vi "Uframe-MNR.vi"() -> ()   [LabVIEW 2010]
uses:
  <vilib>/Platform/TimedLoop/XDataNode/XDataNode.xnode
  <vilib>/Platform/TimedLoop/XDataNode/timing_clust.ctl
  <vilib>/Platform/TimedLoop/XDataNode/nitl_modes.ctl
  <vilib>/Platform/TimedLoop/XDataNode/wakeup.ctl
  <vilib>/Platform/TimedLoop/XDataNode/XDNodeRunTimeDep.lvlib
panel:
  out "Load Cell Constant (N/V)":dbl=44.48
  in  "Load Cell":u16(ring)=1 items=["440 N", "1250 N"]
  in  "Pause @ Load":bool
  in  "Pause @ N":dbl
  out "Disp (mm)":dbl
  out "Load (N)":dbl
  out "Data Point":i32
  in  "Max Load (N)":dbl=600.0 min=0.0 max=1200.0
  out "At Limit":bool
  in  "Rate Multiplier":dbl=1.0
  in  "Pause \nDisplacement":bool
  in  "Stop":bool
  in  "Invert \nDisplacement":bool
  in  "Zero \nDisplacement":bool=TRUE
  in  "Begin":bool
  out "Load vs Disp":cluster{dbl[], dbl[]}(graph)={[-724.1250113144533, -724.195323815552, -724.2656363166506, -724.3359488177492, -724.4062613188479, -724.4765738199465, -724.5468863210451, -724.6171988221438, -724.7461050741579, -724.9218863269045, -725.0976675796511, -725.2851675825808, -725.4492300851442], [-11.89350874713131, -11.896152101474941, -11.894229661847117, -11.89350874707076, -11.890865392620372, -11.895671491596438, -11.895911796524977, -11.899756675680168, -11.899035760801853, -11.90552399441818, -11.907927043887174, -11.905283689458143, -11.914655582386047]}
  out "Disp Vs Time":cluster{dbl[], dbl[]}(graph)={[-724.1250113144533, -724.195323815552, -724.2656363166506, -724.3359488177492, -724.4062613188479, -724.4765738199465, -724.5468863210451, -724.6171988221438, -724.7461050741579, -724.9218863269045, -725.0976675796511, -725.2851675825808, -725.4492300851442], [-11.89350874713131, -11.896152101474941, -11.894229661847117, -11.89350874707076, -11.890865392620372, -11.895671491596438, -11.895911796524977, -11.899756675680168, -11.899035760801853, -11.90552399441818, -11.907927043887174, -11.905283689458143, -11.914655582386047]}
  in  "File Name":string="Test"
  in  "File Path":path=path "C:/cygwin/home/Smarter Materials/Users 2015/Michael Rossol"
  in  "Sample Notes":string
  in  "Displacement \nRate (um/s)":dbl=3.0 min=3.0 max=50.0
  in  "Data Acquisition \nInterval (s)":dbl=1.0 min=0.1 max=10.0 step=0.01 format="%#_3g"
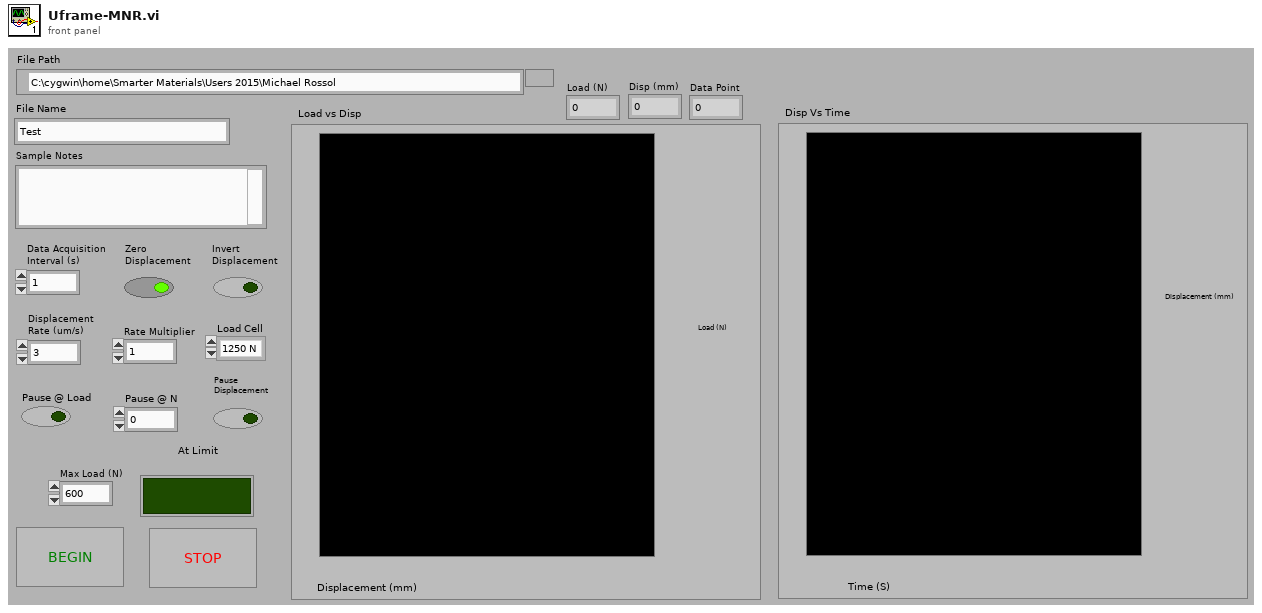
[diagram p1: front panel]
types:
  T1 = typedef "XDNodeRunTimeDep.lvlib/timing_clust.ctl" = cluster{"Expected End [f-1]":u64, "Actual End [f-1]":u64, "Finished Late? [f-1]":bool, "Expected End [i-1]":u64, "Actual End [i-1]":u64, "Finished Late? [i-1]":bool, "Expected Start [i]":u64, "Actual Start [i]":u64, "Expected Start [f]":u64, "Actual Start [f]":u64, "Source Name":string, "Structure Name":string, "Period":i64, "Deadline":i64, "Offset":i64, "Start":i64, "Priority":i32, "Timeout":i32, "Mode":T2, "Wakeup Reason":T3, "Error":errorcluster, "Source Type":string, "Secondary Source Type":string, "Global End Time":u64, "Global Start Time":u64, "Frame Duration":u64, "Iteration Duration":u64, "Assigned CPU":i32, "I/O Scan Engine Mode":u32}
  T2 = typedef "XDNodeRunTimeDep.lvlib/nitl_modes.ctl" = enum32{"No Change", "Process missed periods, maintain original phase", "Discard missed periods, maintain original phase", "Process missed periods, ignore original phase", "Discard missed periods, ignore original phase"}
  T3 = typedef "XDNodeRunTimeDep.lvlib/wakeup.ctl" = enum32{"Normal", "Aborted", "Asynchronous wakeup", "Timing source error", "Timed loop error", "Timeout"}
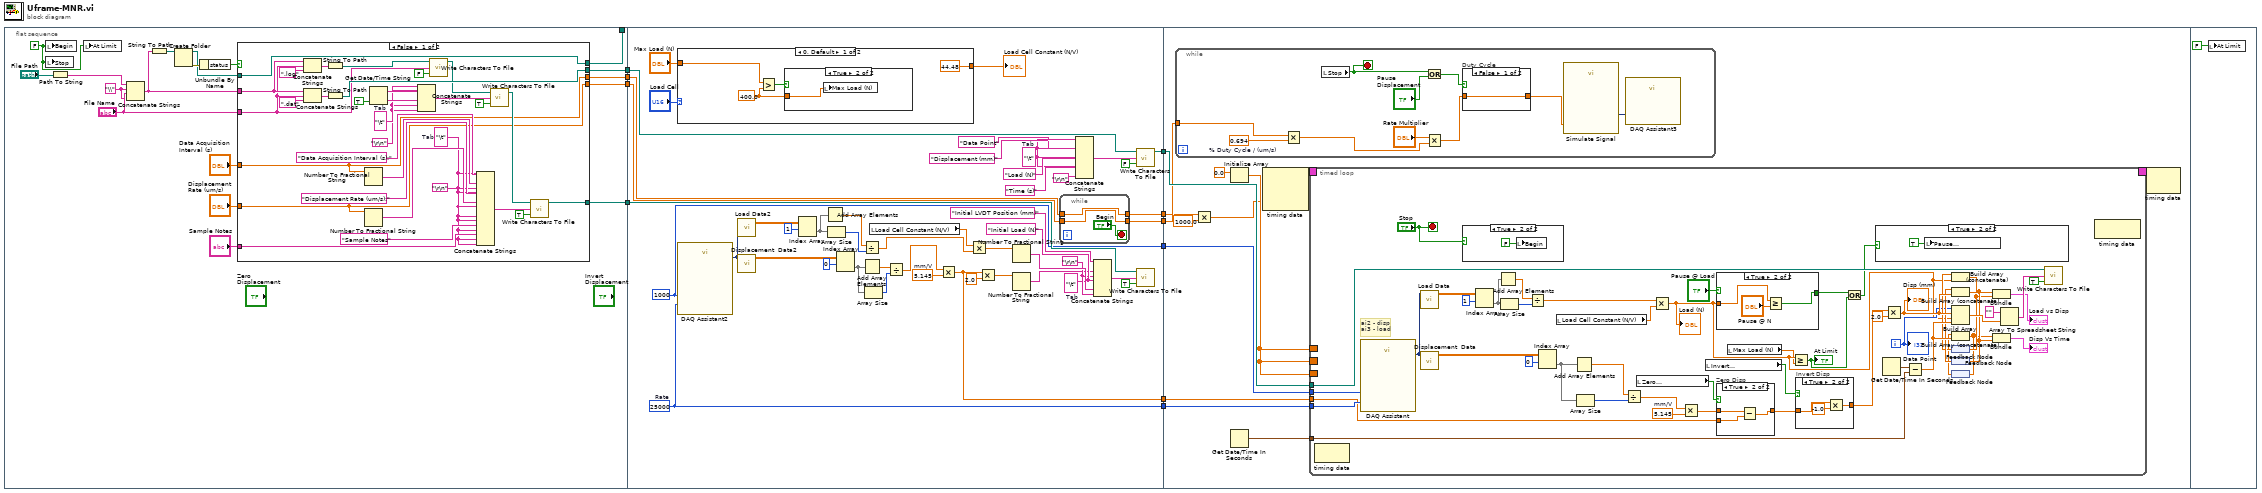
[diagram p0: block diagram]
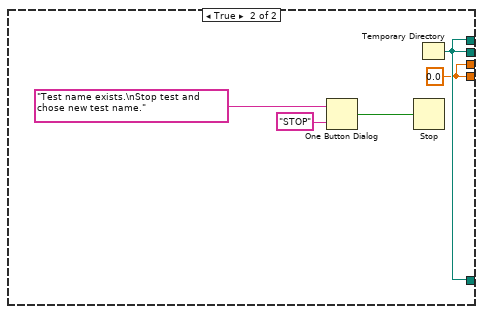
[diagram p2: hidden frame]
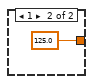
[diagram p4: hidden frame]
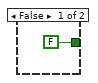
[diagram p5: hidden frame]
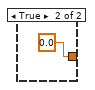
[diagram p10: hidden frame]
diagram:
  n1 = flat-sequence {
    tunnel: [w15] -> w6
    tunnel: [w27] -> w4
    tunnel: [w16] -> w3
    tunnel: [w17] -> w1
    tunnel: [w13] -> _
    tunnel: [w70] -> w10
    tunnel: [w71] -> w9
    tunnel: [w72] -> w8
    tunnel: [w77] -> w7
    tunnel: w6 -> [w91]
    tunnel: [w82] -> w5
    tunnel: w4 -> [w81]
    tunnel: w3 -> [w74]
    tunnel: [w73] -> w2
    tunnel: w1 -> [w75]
    tunnel: w10 -> [w123]
    tunnel: w9 -> [w134]
    tunnel: w8 -> [w133]
    tunnel: w7 -> [w132]
    tunnel: w5 -> [w131]
    tunnel: w2 -> [w130]
    frame #0 {
      w14 = FALSE ("Begin")
      w12 = "\\"
      n2 = local write "Begin"(w14) -> ()
      n3 = local write "Stop"(w14) -> ()
      n4 = Path To String(path="File Path") -> (string=w22:string)
      n5 = local write "At Limit"(w14) -> ()
      n6 = Concatenate Strings(w22, w12, "File Name", w12) -> (w20:string)
      n7 = String To Path(string=w20) -> (path=w24:path)
      n8 = Create Folder(path (use dialog)=w24) -> (created path=w11:path, error out=w23:errorcluster)  [unwired: 2 in, 1 out]
      n9 = Unbundle By Name(w23) -> ("status"=w21:bool)
      n10 = case shown="False" w21 {
        tunnel: [w46 w62] -> w15
        tunnel: "Data Acquisition \nInterval (s)" -> [w41 _]
        tunnel: "Displacement \nRate (um/s)" -> [w42 _]
        tunnel: "Sample Notes" -> [w38 _]
        tunnel: [w43 w62] -> w27
        tunnel: [w42 w61] -> w16
        tunnel: [w41 w61] -> w17
        tunnel: w20 -> [w31 _]
        tunnel: "File Name" -> [w30 _]
        tunnel: [w29 w62] -> w13
        tunnel: w11 -> [w29 _]
        frame False {
          w40 = "\t"  # Tab
          w37 = "\r\n"
          w56 = "\t"  # Tab
          w51 = "\r\n"
          n11 = Concatenate Strings(w31, w30, ".log") -> (w33:string)
          n12 = Concatenate Strings(w31, w30, ".dat") -> (w44:string)
          n13 = String To Path(string=w33) -> (path=w32:path)
          n14 = String To Path(string=w44) -> (path=w43:path)
          n15 = Number To Fractional String(number=w41) -> (F-format string=w49:string)  [unwired: 3 in]
          n16 = Number To Fractional String(number=w42) -> (F-format string=w47:string)  [unwired: 3 in]
          n17 = Get Date/Time String(want seconds? (F)=TRUE) -> (date string=w59:string, time string=w58:string)  [unwired: 2 in]
          n18 = Concatenate Strings(w51, w59, w56, w58, w51, w51) -> (w60:string)
          n19 = call <vilib>:"Write Characters To File.vi"("append to file? (new file:F)"=FALSE, "character string"=w30, "file path (dialog if empty)"=w32) -> ("new file path (Not A Path if cancelled)"=w36:path)  [unwired: 2 in]
          n20 = Concatenate Strings("Data Acquisition Interval (s):", w40, w49, w37, "Displacement Rate (um/s):", w40, w47, w37, w40, w37, w37, "Sample Notes", w37, w38, w37, w37) -> (w52:string)
          n21 = call <vilib>:"Write Characters To File.vi"("append to file? (new file:F)"=TRUE, "character string"=w60, "file path (dialog if empty)"=w36) -> ("new file path (Not A Path if cancelled)"=w54:path)  [unwired: 2 in]
          n22 = call <vilib>:"Write Characters To File.vi"("append to file? (new file:F)"=TRUE, "character string"=w52, "file path (dialog if empty)"=w54) -> ("new file path (Not A Path if cancelled)"=w46:path)  [unwired: 2 in]
        }
        frame True {
          w61 = 0.0 ("Displacement Rate (um/s)")
          n23 = One Button Dialog(message="Test name exists.\nStop test and chose new test name.", button name ("OK")="STOP") -> (true=w63:bool)
          n24 = Stop(stop? (T)=w63) -> ()
          n25 = Temporary Directory() -> (w62:path)
        }
      }
    }
    frame #1 {
      w72 = 1000 ("number of samples")
      w84 = "\t"  # Tab
      w95 = "\r\n"
      w93 = "\t"  # Tab
      w109 = 5.145  # mm/V
      w71 = 25000  # Rate
      n26 = case shown="0, Default" "Load Cell" {
        tunnel: [44.48 125.0] -> w68
        tunnel: "Max Load (N)" -> [w114 _]
        frame 0, Default {
          w113 = 400.0 ("y")
          n27 = Greater?(x=w114, y=w113) -> (0:w115:bool)
          n28 = case shown="True" w115 {
            tunnel: w113 -> [_ w117]
            frame False {
            }
            frame True {
              n29 = local write "Max Load (N)"(w117) -> ()
            }
          }
        }
        frame 1 {
        }
      }
      "Load Cell Constant (N/V)" <- w68
      n30 = call "DAQ Assistant2"("rate"=w71, "number of samples"=w72) -> ("data"=w100:dynamicdata)  [unwired: 15 in, 2 out]
      n31 = call "Load Data2"("Dynamic Data Type"=w100) -> ("Array"=w101:dbl[][])  [unwired: 3 in]
      n32 = call "Displacement  Data2"("Dynamic Data Type"=w100) -> ("Array"=w104:dbl[][])  [unwired: 3 in]
      n33 = Index Array(array=w101, index (row)=1) -> (element=w112:dbl[])  [unwired: 1 in]
      n34 = Add Array Elements(numeric array=w112) -> (sum=w110:dbl)
      n35 = Array Size(array=w112) -> (size(s)=w111:i32)
      n36 = Index Array(array=w104, index (row)=0) -> (element=w105:dbl[])  [unwired: 1 in]
      n37 = Divide(x=w110, y=w111) -> (x/y=w79:dbl)
      n38 = Add Array Elements(numeric array=w105) -> (sum=w106:dbl)
      n39 = Array Size(array=w105) -> (size(s)=w107:i32)
      n40 = local read "Load Cell Constant (N/V)"() -> (w69:dbl)
      n41 = Divide(x=w106, y=w107) -> (x/y=w108:dbl)
      n42 = Multiply(x=w108, y=w109) -> (x*y=w77:dbl)
      n43 = Multiply(x=w69, y=w79) -> (x*y=w80:dbl)
      n44 = Multiply(x=w77, y=2.0) -> (x*y=w78:dbl)
      n45 = Number To Fractional String(number=w80) -> (F-format string=w97:string)  [unwired: 3 in]
      n46 = Number To Fractional String(number=w78) -> (F-format string=w94:string)  [unwired: 3 in]
      n47 = while {
        tunnel: w74 -> [w120]
        tunnel: [w120] -> w73
        tunnel: [w119] -> w70
        tunnel: w75 -> [w119]
        stop <- "Begin" stop-if-true
      }
      n48 = Concatenate Strings("Data Point", w84, "Displacement (mm)" ("Substring"), w84, "Load (N)", w84, "Time (s)" ("string"), w84, "\r\n") -> (w89:string)
      n49 = Concatenate Strings("Initial LVDT Position (mm)", w93, w94, w95, "Initial Load (N)", w93, w97, w95) -> (w98:string)
      n50 = call <vilib>:"Write Characters To File.vi"("append to file? (new file:F)"=FALSE, "character string"=w89, "file path (dialog if empty)"=w81) -> ("new file path (Not A Path if cancelled)"=w82:path)  [unwired: 2 in]
      n51 = call <vilib>:"Write Characters To File.vi"("append to file? (new file:F)"=TRUE, "character string"=w98, "file path (dialog if empty)"=w91) -> ()  [unwired: 2 in, 1 out]
    }
    frame #2 {
      n52 = while {
        tunnel: w130 -> [w211]
        stop <- w204 stop-if-true
        w205 = 0.694  # % Duty Cycle / (um/s)
        n53 = Multiply(x=w211, y=w205) -> (x*y=w208:dbl)
        n54 = local read "Stop"() -> (w204:bool)
        n55 = Or(x=w204, y="Pause \nDisplacement") -> (x .or. y?=w210:bool)
        n56 = Multiply(x="Rate Multiplier", y=w208) -> (x*y=w207:dbl)
        n57 = case "Duty Cycle" shown="False" w210 {
          tunnel: [w214 0.0 ("Duty Cycle (%)")] -> w212
          tunnel: w207 -> [w214 _]
          frame False {
          }
          frame True {
          }
        }
        n58 = call "Simulate Signal"("Duty Cycle (%)"=w212) -> ("Square"=w213:dynamicdata)  [unwired: 13 in, 1 out]
        n59 = call "DAQ Assistant3"("data"=w213) -> ()  [unwired: 16 in, 3 out]
      }
      n60 = Multiply(x=w123, y=1000.0) -> (x*y=w124:dbl)
      n61 = Get Date/Time In Seconds() -> (seconds since 1Jan1904=w127:timestamp)
      n62 = Initialize Array(0.0) -> (w128:dbl[])  [unwired: 1 in]
      n63 = node-c288(w124) -> (w126:T1)  [unwired: 2 in]
      n64 = timed-loop {
        tunnel: w133 -> [w166]
        tunnel: w134 -> [w165]
        tunnel: w132 -> [w157]
        tunnel: w127 -> [w161]
        tunnel: w131 -> [w160]
        border: w128 -> [_]
        border: w128 -> [_]
        border: w128 -> [_]
        timing: w126 -> [_]
        timing-out: [_] -> w125
        i -> [w143]
        stop <- "Stop" stop-if-true
        w164 = 5.145  # mm/V
        # "ai2 - disp\nai3 - load"
        n65 = node-c288() -> ()  [unwired: 1 in, 1 out]
        n66 = call "DAQ Assistant"("rate"=w165, "number of samples"=w166) -> ("data"=w163:dynamicdata)  [unwired: 15 in, 2 out]
        n67 = call "Load Data"("Dynamic Data Type"=w163) -> ("Array"=w178:dbl[][])  [unwired: 3 in]
        n68 = call "Displacement  Data"("Dynamic Data Type"=w163) -> ("Array"=w175:dbl[][])  [unwired: 3 in]
        n69 = case shown="True" "Stop" {
          frame False {
          }
          frame True {
            n70 = local write "Begin"(FALSE ("Begin")) -> ()
          }
        }
        n71 = Index Array(array=w178, index (row)=1) -> (element=w167:dbl[])  [unwired: 1 in]
        n72 = Add Array Elements(numeric array=w167) -> (sum=w169:dbl)
        n73 = Array Size(array=w167) -> (size(s)=w168:i32)
        n74 = Divide(x=w169, y=w168) -> (x/y=w154:dbl)
        n75 = Index Array(array=w175, index (row)=0) -> (element=w173:dbl[])  [unwired: 1 in]
        n76 = local read "Load Cell Constant (N/V)"() -> (w136:dbl)
        n77 = Add Array Elements(numeric array=w173) -> (sum=w172:dbl)
        n78 = Array Size(array=w173) -> (size(s)=w171:i32)
        n79 = Divide(x=w172, y=w171) -> (x/y=w170:dbl)
        n80 = local read "Zero \nDisplacement"() -> (w155:bool)
        n81 = Multiply(x=w154, y=w136) -> (x*y=w138:dbl)
        "Load (N)" <- w138
        n82 = Multiply(x=w170, y=w164) -> (x*y=w159:dbl)
        n83 = local read "Invert \nDisplacement"() -> (w156:bool)
        n84 = case shown="True" "Pause @ Load" {
          tunnel: w138 -> [_ w186]
          tunnel: [FALSE w185] -> w137
          frame False {
          }
          frame True {
            n85 = Greater Or Equal?(x=w186, y="Pause @ N") -> (x >= y?=w185:bool)
          }
        }
        n86 = case "Zero Disp" shown="True" w155 {
          tunnel: w157 -> [_ w199]
          tunnel: w159 -> [w196 w198]
          tunnel: [w196 w197] -> w158
          frame False {
          }
          frame True {
            n87 = Subtract(x=w198, y=w199) -> (x-y=w197:dbl)
          }
        }
        n88 = local read "Max Load (N)"() -> (w135:dbl)
        n89 = Greater Or Equal?(x=w138, y=w135) -> (x >= y?=w140:bool)
        "At Limit" <- w140
        n90 = case "Invert Disp" shown="True" w156 {
          tunnel: w158 -> [w192 w195]
          tunnel: [w192 w194] -> w152
          frame False {
          }
          frame True {
            n91 = Multiply(x=w195, y=-1.0) -> (x*y=w194:dbl)
          }
        }
        n92 = Or(x=w137, y=w140) -> (x .or. y?=w141:bool)
        n93 = case shown="True" w141 {
          frame False {
          }
          frame True {
            n94 = local write "Pause \nDisplacement"(TRUE ("Pause \nDisplacement")) -> ()
          }
        }
        n95 = Get Date/Time In Seconds() -> (seconds since 1Jan1904=w174:timestamp)
        n96 = Multiply(x=w152, y=2.0) -> (x*y=w151:dbl)
        "Disp (mm)" <- w151
        n97 = Subtract(x=w174, y=w161) -> (x-y=w162:dbl)
        n98 = Build Array(w143, w151, w138, w162) -> (w180:dbl[])
        n99 = feedback #1() -> (w146:dbl[])
        n100 = Build Array (concatenate)(w146, w138) -> (w147:dbl[])
        n101 = feedback-in #1(w147) -> ()
        n102 = feedback #2() -> (w148:dbl[])
        n103 = Build Array (concatenate)(w148, w151) -> (w149:dbl[])
        n104 = feedback-in #2(w149) -> ()
        n105 = feedback #3() -> (w144:dbl[])
        n106 = Build Array (concatenate)(w144, w162) -> (w145:dbl[])
        n107 = feedback-in #3(w145) -> ()
        n108 = Bundle(w149, w147) -> (→"Load vs Disp":cluster{dbl[], dbl[]})  [unwired: 1 in]
        n109 = Bundle(w145, w149) -> (→"Disp Vs Time":cluster{dbl[], dbl[]})  [unwired: 1 in]
        n110 = Array To Spreadsheet String(array=w180, 3:"" ("format string")) -> (spreadsheet string=w182:string)  [unwired: 1 in]
        n111 = call <vilib>:"Write Characters To File.vi"("append to file? (new file:F)"=TRUE, "character string"=w182, "file path (dialog if empty)"=w160) -> ()  [unwired: 2 in, 1 out]
        n112 = node-c288() -> ()  [unwired: 1 in, 1 out]
        "Data Point" <- w143
      }
      n113 = node-c288(w125) -> ()  [unwired: 1 out]
    }
    frame #3 {
      n114 = local write "At Limit"(FALSE ("Begin")) -> ()
    }
  }
